vi "Byte Buffer.Read (1D U8).vi"(8 "error in (no error)":errorcluster, 9 "count":i32, 10 "buffer offset":i32, 11 "Byte Buffer in":refnum<class "Byte Buffer.lvclass">) -> (0 "error out":errorcluster, 1 "value":u8[](array[numeric]), 3 "Byte Buffer out":refnum<class "Byte Buffer.lvclass">)   [LabVIEW 2016, in "VeriStand Data.lvlib" / "Byte Buffer.lvclass"]
doc: "Reads <B>count</B> elements of data from the provided <B>Byte Buffer</B> at location <B>buffer offset</B> in the format of the data type specified."
uses:
  Byte Buffer.lvclass
  Byte Buffer.lvclass/Byte Buffer.ctl
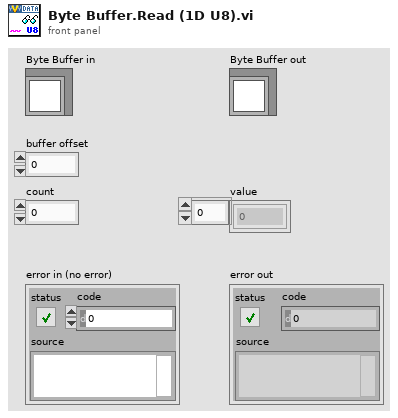
[diagram p1: front panel]
types:
  T1 = enum16{"big-endian, network order", "native, host order", "little-endian"}
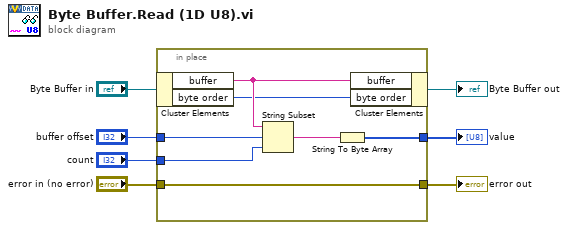
[diagram p0: block diagram]
diagram:
  n1 = in-place {
    in-place-border: "buffer offset" -> [w14]
    in-place-border: "error in (no error)" -> [w8]
    in-place-border: [w8] -> w5
    in-place-border: [w9] -> w4
    in-place-border: "count" -> [w11]
    n2 = in-place-cluster #1("Byte Buffer in") -> ("buffer"=w13:string, "byte order"=w12:T1)
    n3 = String Subset(string=w13, offset (0)=w14, length (rest)=w11) -> (substring=w10:string)
    n4 = String To Byte Array(string=w10) -> (unsigned byte array=w9:u8[])
    n5 = in-place-cluster #1("buffer"=w13, "byte order"=w12) -> (→"Byte Buffer out":refnum<class "Byte Buffer.lvclass">)
  }
  "value" <- w4
  "error out" <- w5
